vi "LVClass_Camera dtor.vi"(0 "Camera in":refnum<class "Camera.lvclass">, 11 "error in (no error)":errorcluster) -> (4 "Camera out":refnum<class "Camera.lvclass">, 15 "error out":errorcluster)   [LabVIEW 2020, in "Camera.lvclass"]
doc: "Camera destructor.\n\n--------------------------------------------------------------------------------\n\n<B>CameraIn </B> : Camera object.\n<B>CameraOut </B> : Camera object.\n<B>ErrorIn </B> : Error\n<B>ErrorOut </B> : Error\n\n--------------------------------------------------------------------------------"
uses:
  Camera.lvclass
  Camera.lvclass/Camera.ctl
  Image.lvclass
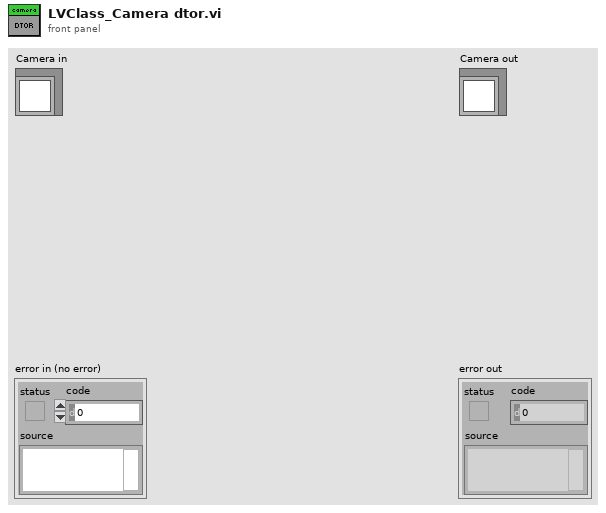
[diagram p1: front panel]
types:
  T1 = typedef "Handle creation.ctl" = enum16{"By ctor", "By write function"}
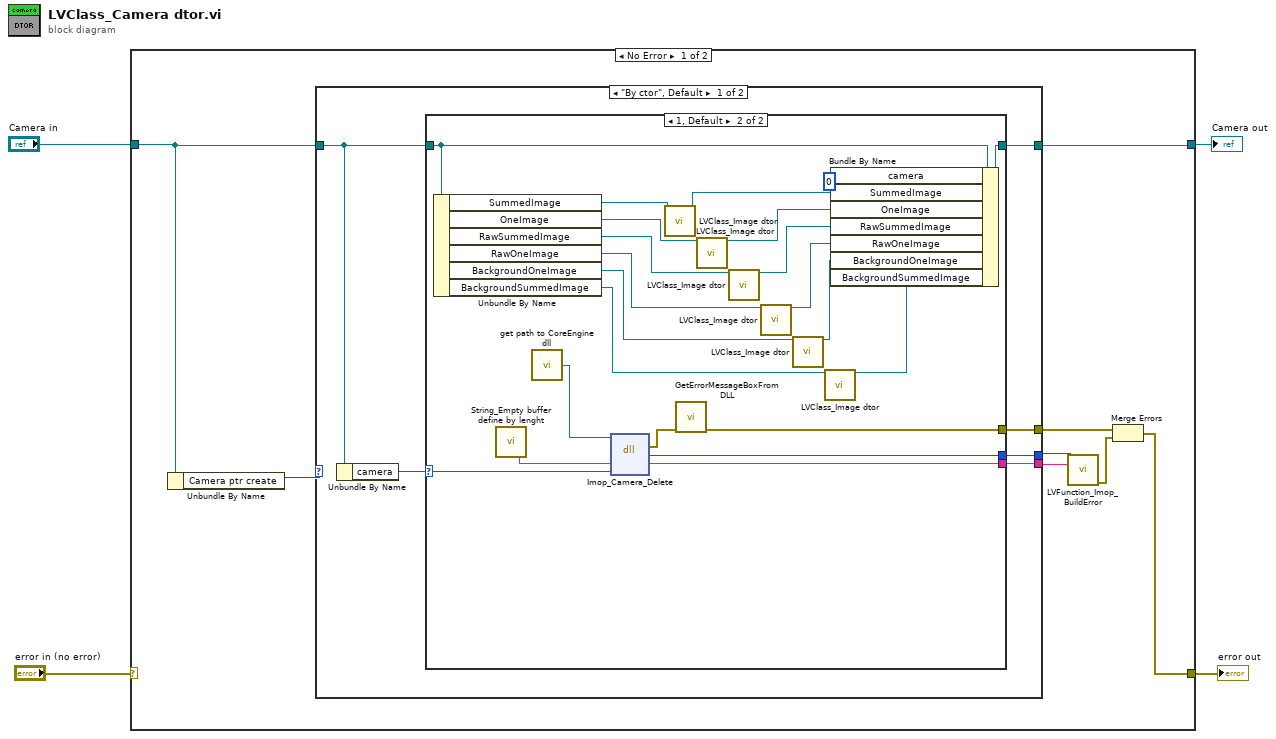
[diagram p0: block diagram]
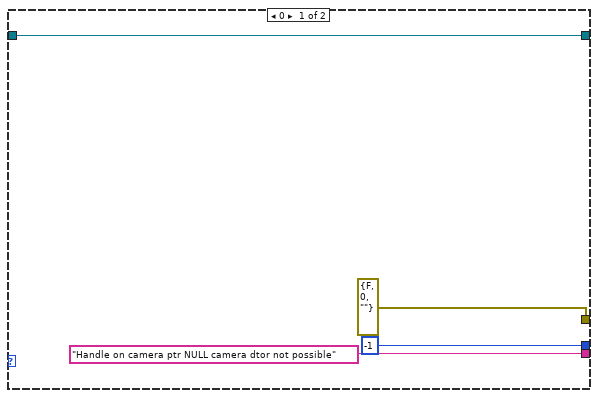
[diagram p2: hidden frame]
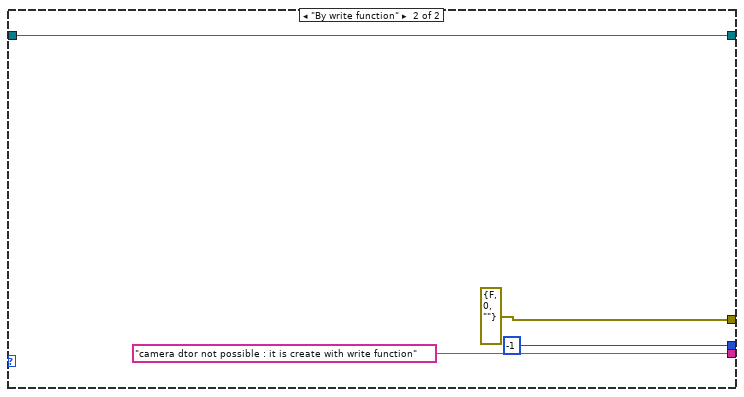
[diagram p3: hidden frame]
diagram:
  n1 = case shown="No Error" "error in (no error)" {
    selector: "error in (no error)" -> [_ w50]
    tunnel: [w5 w50] -> w3
    tunnel: [w8 w49] -> w1
    tunnel: "Camera in" -> [w9 w49]
    frame No Error {
      n2 = Unbundle By Name(w9) -> ("Camera ptr create"=w10:T1)
      n3 = case shown="\"By ctor\", Default" w10 {
        tunnel: [w18 w48] -> w8
        tunnel: [w16 -1] -> w12
        tunnel: [w15 "camera dtor not possible : it is create with write function" ("message")] -> w11
        tunnel: w9 -> [w14 w48]
        tunnel: [w13 errorcluster {"status"=FALSE, "code"=0, "source"=""} ("error OUT")] -> w7
        frame "By ctor", Default {
          n4 = Unbundle By Name(w14) -> ("camera"=w17:i32)
          n5 = case shown="1, Default" w17 {
            selector: w17 -> [_ w41]
            tunnel: w14 -> [w22 w36]
            tunnel: [w22 w44] -> w18
            tunnel: [-1 w39] -> w16
            tunnel: ["Handle on camera ptr NULL camera dtor not possible" ("message") w40] -> w15
            tunnel: [errorcluster {"status"=FALSE, "code"=0, "source"=""} ("error OUT") w29] -> w13
            frame 0 {
            }
            frame 1, Default {
              n6 = Unbundle By Name(w36) -> ("SummedImage"=w35:refnum<class "Image.lvclass">, "OneImage"=w34:refnum<class "Image.lvclass">, "RawSummedImage"=w33:refnum<class "Image.lvclass">, "RawOneImage"=w32:refnum<class "Image.lvclass">, "BackgroundOneImage"=w31:refnum<class "Image.lvclass">, "BackgroundSummedImage"=w30:refnum<class "Image.lvclass">)
              n7 = call "String_Empty buffer define by lenght.vi"() -> ("Empty buffer"=w42:string)  [unwired: 1 in]
              n8 = call "get path to CoreEngine dll.vi"() -> ("path to c_interface_vc100.dll"=w38:path)  [unwired: 12 in, 3 out]
              n9 = dll-call lib="D:/soft/HASO_v3/SVN_trunk/ImOpCoreEngine4_LV2011/DLLs/c_interface_vc100.dll" fn="Imop_Camera_Delete"(path in=w38, "message"=w42, "objet"=w41) -> (error out=w37:errorcluster, "return type"=w39:i32, "message"=w40:string)  [unwired: 3 in, 1 out]
              n10 = call "LVClass_Image dtor.vi"("Image in"=w35) -> ("Image out"=w28:refnum<class "Image.lvclass">)  [unwired: 13 in, 1 out]
              n11 = call "GetErrorMessageBoxFromDLL.vi"("error IN"=w37) -> ("error OUT"=w29:errorcluster)  [unwired: 10 in]
              n12 = call "LVClass_Image dtor.vi"("Image in"=w34) -> ("Image out"=w27:refnum<class "Image.lvclass">)  [unwired: 13 in, 1 out]
              n13 = call "LVClass_Image dtor.vi"("Image in"=w33) -> ("Image out"=w26:refnum<class "Image.lvclass">)  [unwired: 13 in, 1 out]
              n14 = call "LVClass_Image dtor.vi"("Image in"=w32) -> ("Image out"=w25:refnum<class "Image.lvclass">)  [unwired: 13 in, 1 out]
              n15 = call "LVClass_Image dtor.vi"("Image in"=w31) -> ("Image out"=w24:refnum<class "Image.lvclass">)  [unwired: 13 in, 1 out]
              n16 = call "LVClass_Image dtor.vi"("Image in"=w30) -> ("Image out"=w23:refnum<class "Image.lvclass">)  [unwired: 13 in, 1 out]
              n17 = Bundle By Name(cluster=w36, "camera"=0, "SummedImage"=w28, "OneImage"=w27, "RawSummedImage"=w26, "RawOneImage"=w25, "BackgroundOneImage"=w24, "BackgroundSummedImage"=w23) -> (w44:refnum<class "Camera.lvclass">)
            }
          }
        }
        frame "By write function" {
        }
      }
      n18 = call "LVFunction_Imop_BuildError.vi"("code"=w12, "String to Prepend to source (\"\")"=w11) -> ("error out"=w6:errorcluster)  [unwired: 13 in]
      n19 = Merge Errors(w7, w6) -> (w5:errorcluster)
    }
    frame Error {
    }
  }
  "error out" <- w3
  "Camera out" <- w1
